vi "Splitting Array(SubVI).vi"(8 "array":dbl[][](array[numeric])) -> (0 "array of all":dbl[][][](array[numeric]))   [LabVIEW 2016]
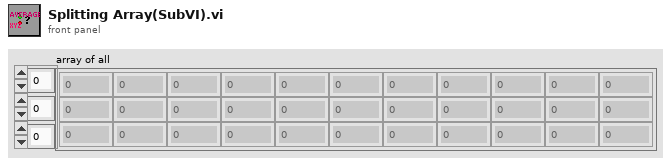
[diagram p1: front panel]
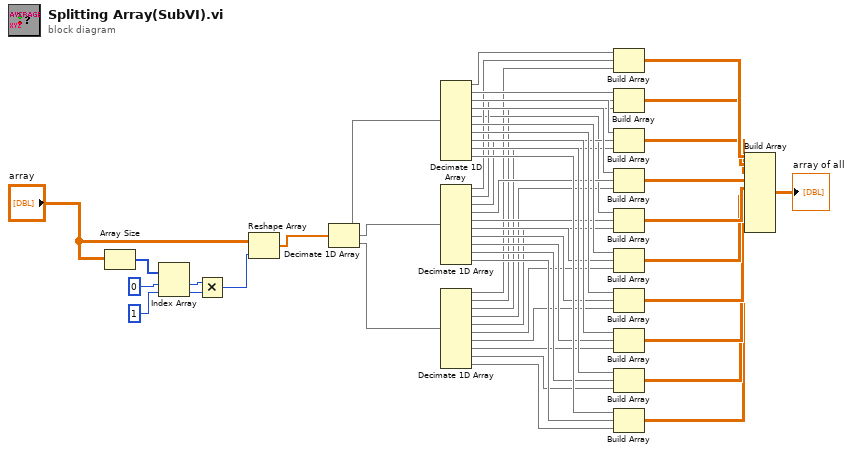
[diagram p0: block diagram]
diagram:
  n1 = Array Size(array="array") -> (size(s)=w52:i32[])
  n2 = Index Array(array=w52, index #1=0 ("index"), index #2=1 ("index")) -> (element #1=w49:i32, element #2=w48:i32)
  n3 = Multiply(x=w49, y=w48) -> (x*y=w1:i32)
  n4 = Reshape Array("array", w1) -> (w46:dbl[])
  n5 = Decimate 1D Array(w46) -> (w45:dbl[], w35:dbl[], w34:dbl[])
  n6 = Decimate 1D Array(w45) -> (w44:dbl[], w43:dbl[], w42:dbl[], w41:dbl[], w18:dbl[], w40:dbl[], w39:dbl[], w38:dbl[], w37:dbl[], w36:dbl[])
  n7 = Decimate 1D Array(w35) -> (w33:dbl[], w32:dbl[], w20:dbl[], w19:dbl[], w31:dbl[], w30:dbl[], w29:dbl[], w28:dbl[], w27:dbl[], w26:dbl[])
  n8 = Decimate 1D Array(w34) -> (w13:dbl[], w14:dbl[], w15:dbl[], w16:dbl[], w17:dbl[], w21:dbl[], w22:dbl[], w23:dbl[], w24:dbl[], w25:dbl[])
  n9 = Build Array(w44, w33, w13) -> (w12:dbl[][])
  n10 = Build Array(w43, w32, w14) -> (w11:dbl[][])
  n11 = Build Array(w42, w20, w15) -> (w10:dbl[][])
  n12 = Build Array(w41, w19, w16) -> (w9:dbl[][])
  n13 = Build Array(w18, w31, w17) -> (w8:dbl[][])
  n14 = Build Array(w40, w30, w21) -> (w7:dbl[][])
  n15 = Build Array(w39, w29, w22) -> (w6:dbl[][])
  n16 = Build Array(w38, w28, w23) -> (w5:dbl[][])
  n17 = Build Array(w37, w27, w24) -> (w4:dbl[][])
  n18 = Build Array(w36, w26, w25) -> (w3:dbl[][])
  n19 = Build Array(w12, w11, w10, w9, w8, w7, w6, w5, w4, w3) -> (→"array of all":dbl[][][])
